vi "VISA_ReadAndSave_8CHparalelos COM BUFFER DE LEITURA.vi"() -> ()   [LabVIEW 2019]
uses:
  813f916b-c519-439e-9418-14bd48b6d342.vi
  <vilib>/Instr/_visa.llb/VISA Configure Serial Port (Instr).vi
  <vilib>/Analysis/Matrix/Comparison/Not Equal/Not Equal.vi
  <vilib>/Analysis/Matrix/Comparison/Not Equal/Not Equal - RM,RM.vi
panel:
  in  "Tamanho do Buffer (leitura/plot)":i32=10
  out "loop time (ms)":dbl format="%.2f"
  out "Plot 7":dbl[](graph)
  out "Plot 6":dbl[](graph)
  out "Plot 5":dbl[](graph)
  out "Plot 4":dbl[](graph)
  out "Plot 3":dbl[](graph)
  out "Plot 2":dbl[](graph)
  out "Status Arquivo":errorcluster
  in  "file name":string
  out "Plot 1":dbl[](graph)
  out "Plot 0":dbl[](graph)
  out "Status Leitura":errorcluster
  out "Conversão Numérica":dbl[](array[numeric])
  out "Prévia da Leitura":string
  out "Status USB":errorcluster
  in  "Salvar Registro":bool
  in  "Gravando":bool
  in  "baud rate (115200)":u32=115200 caption="baud rate (9600)"
  in  "data bits (8)":u8=8 min=5 max=8 step=1
  in  "VISA resource name":refnum<visa-resource-name>="COM3"
  # "Controle de Salvamento"
  # "Log de Erros"
  # "Conversão Para Inteiro"
  # "Resultado da Leitura"
  # "Controle da porta Serial USB"
  # "Controle da Leitura"
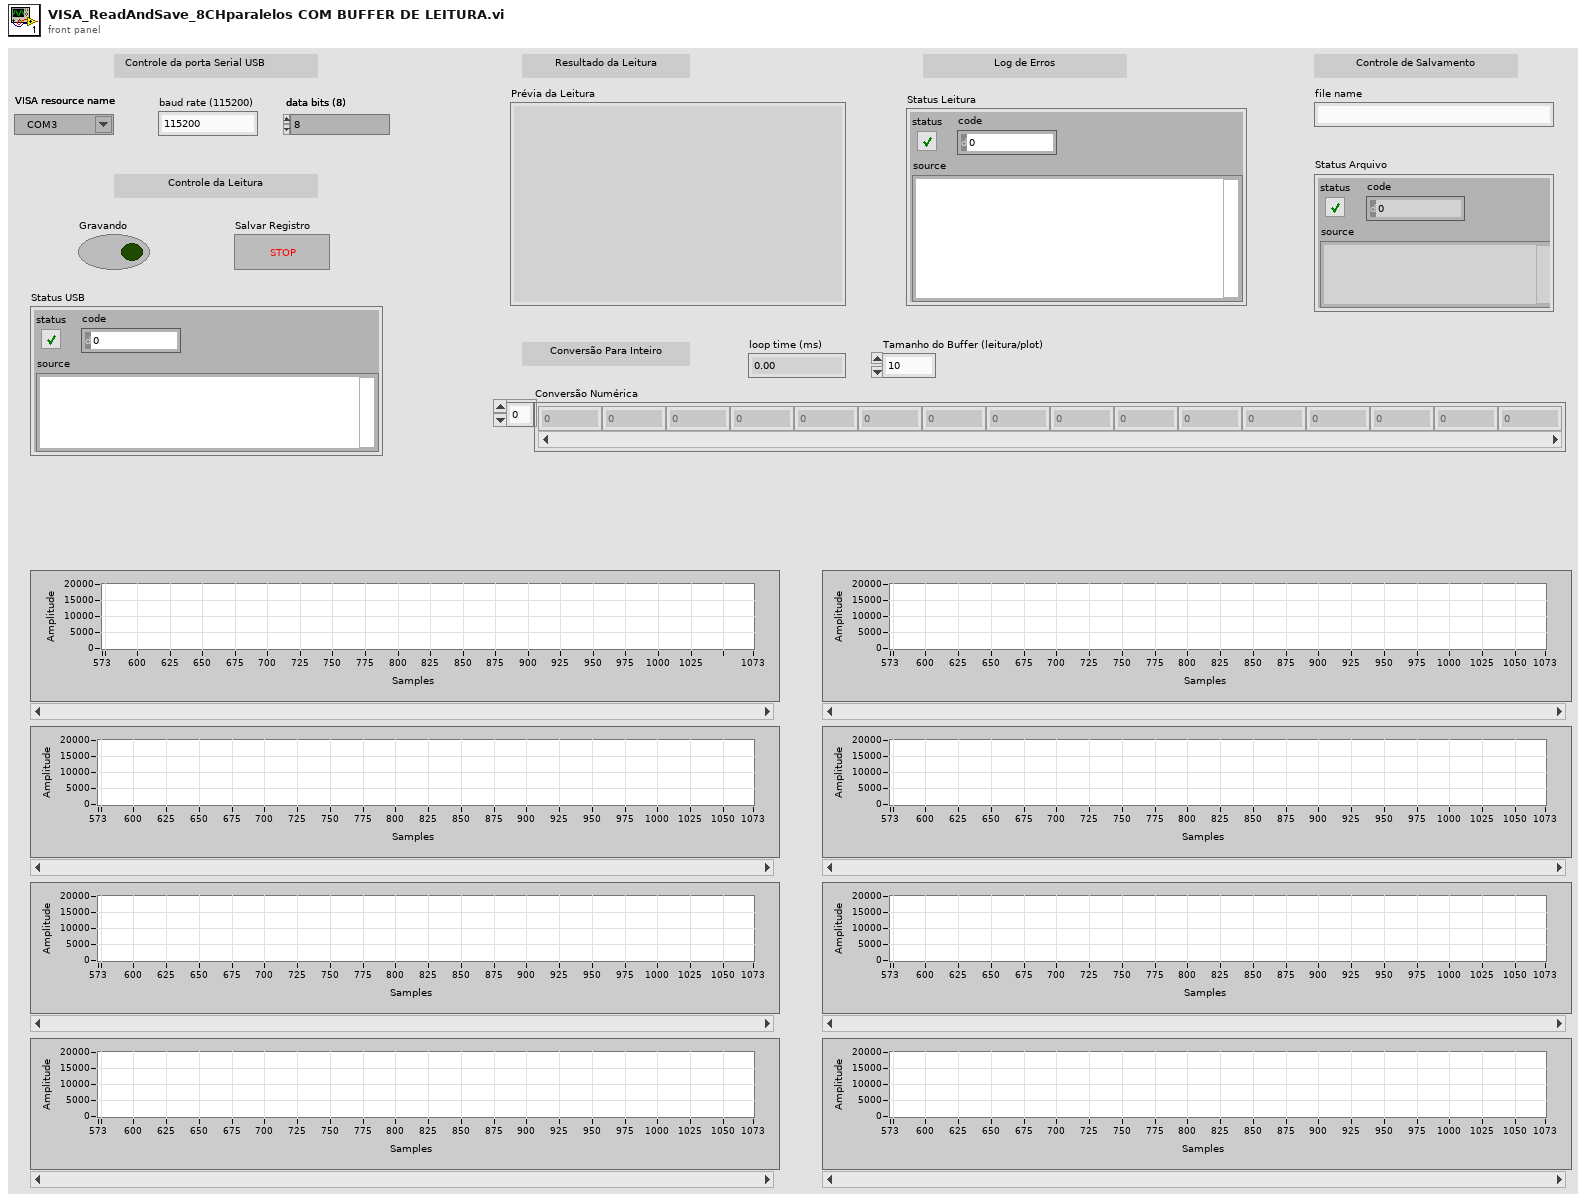
[diagram p1: front panel]
types:
  T1 = typedef "NI_Matrix.lvlib/RealMatrix.ctl" = dbl[][]
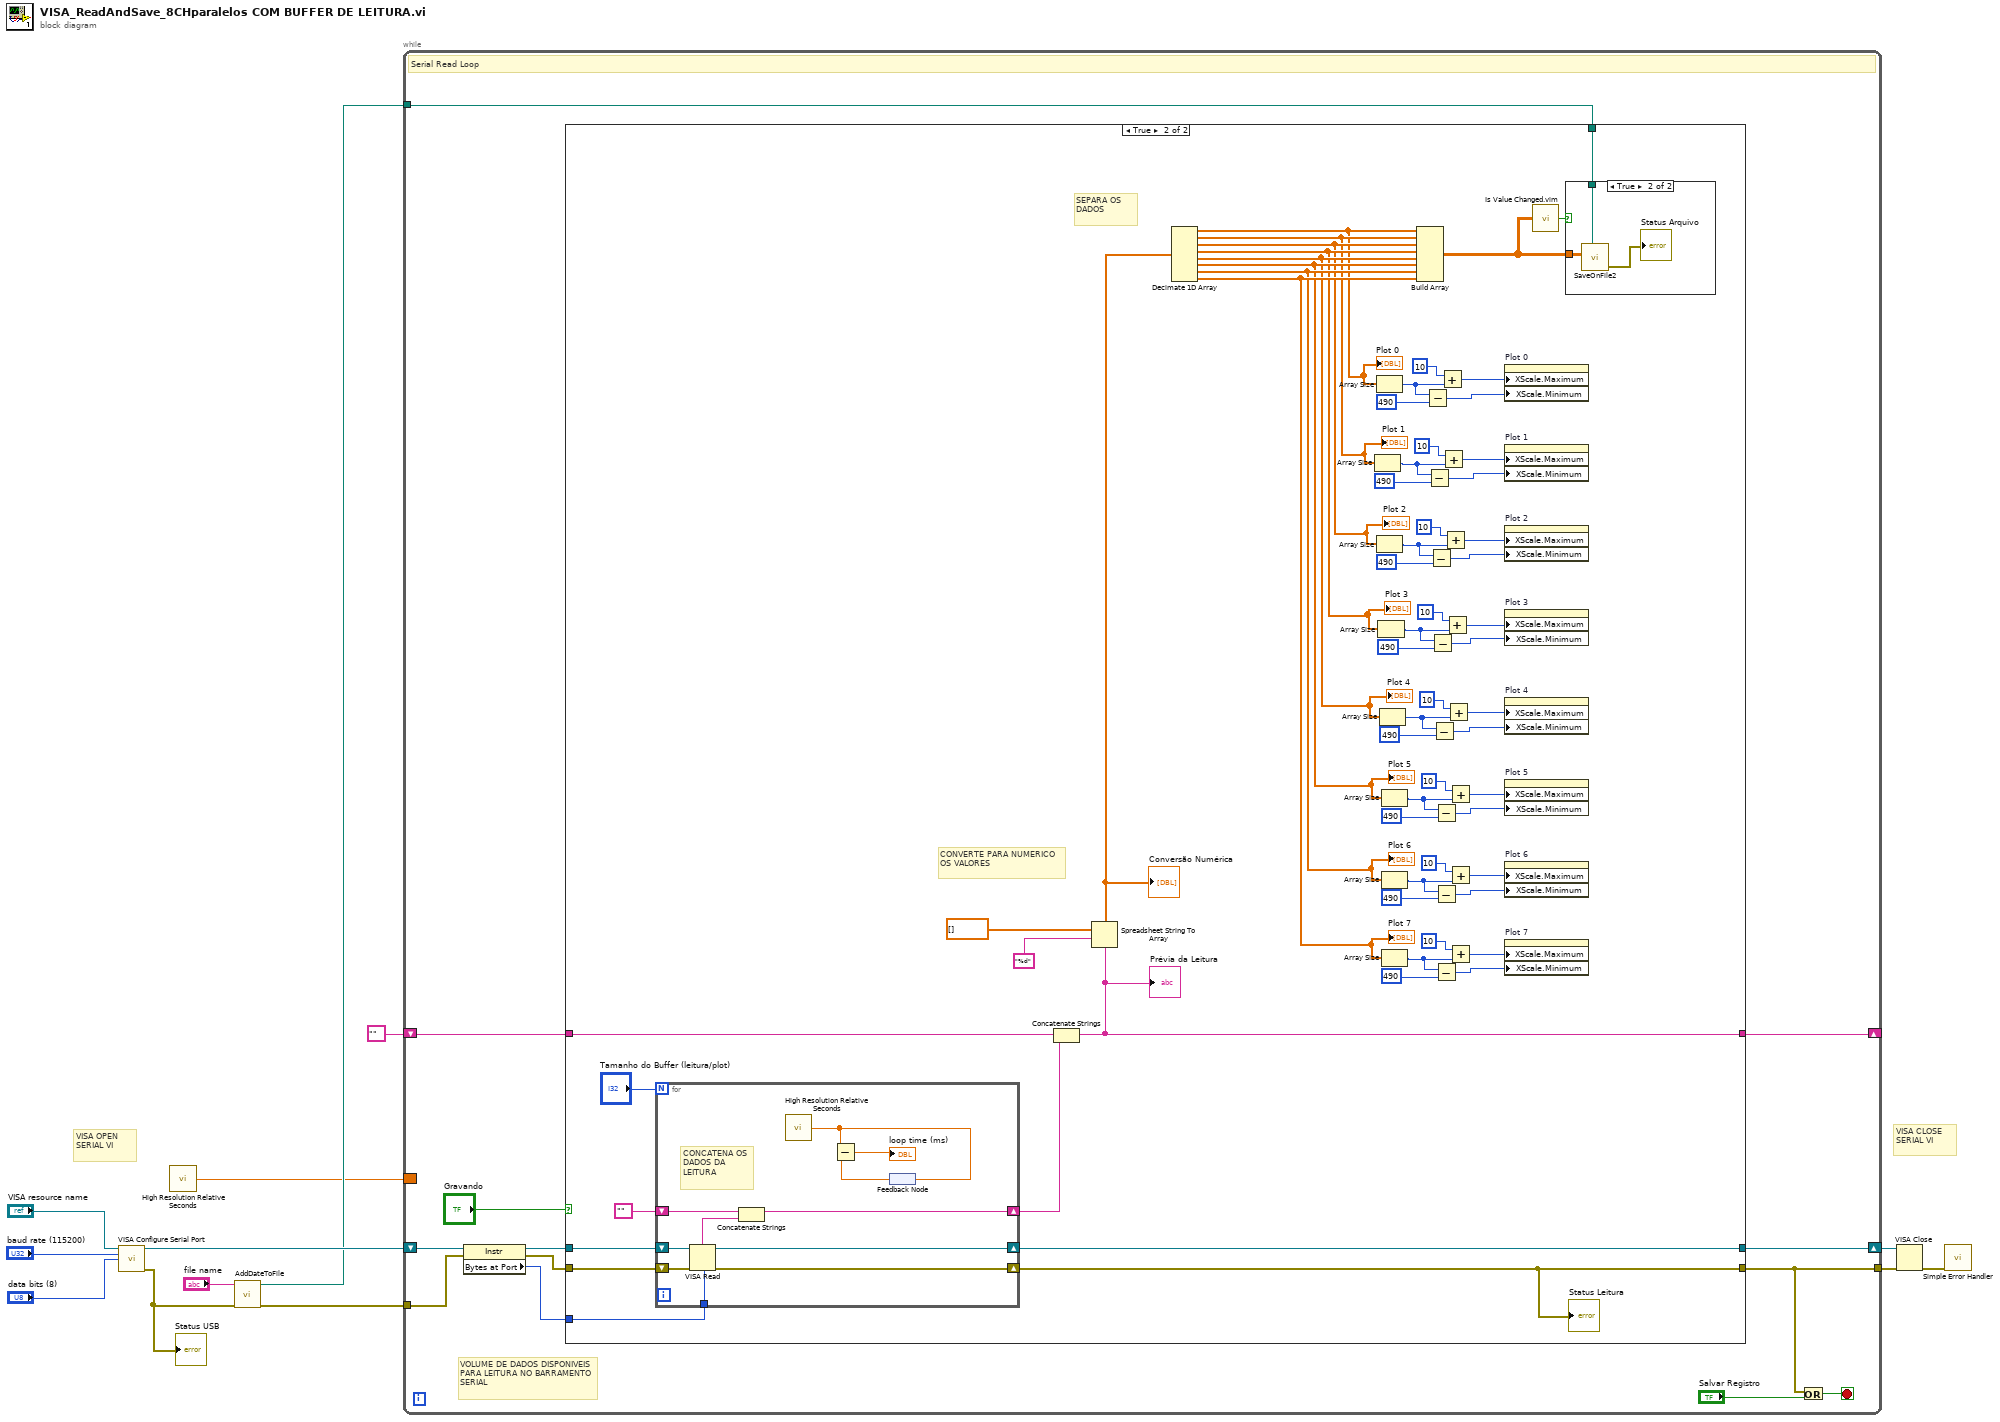
[diagram p0: block diagram]
diagram:
  # "VISA OPEN SERIAL VI"
  # "VISA CLOSE SERIAL VI"
  n1 = call-poly "VISA Configure Serial Port"("VISA resource name"="VISA resource name", "baud rate (9600)"="baud rate (115200)", "data bits (8)"="data bits (8)") -> ("VISA resource name out"=w11:refnum<visa-resource-name>, "error out"=w4:errorcluster)  [unwired: 11 in]
  "Status USB" <- w4
  n2 = call <vilib>:"High Resolution Relative Seconds.vi"() -> ("relative seconds"=w2:dbl)
  n3 = call "AddDateToFile.vi"("error in (no error)"=w4, "file name"="file name") -> ("error out"=w5:errorcluster, "new file path (Not A Path if cancelled)"=w3:path)  [unwired: 8 in]
  n4 = while {
    tunnel: w5 -> [w18]
    tunnel: [w24] -> w12
    shift-right: [w23] -> w10
    shift-left: w11 -> [w21]
    tunnel: w3 -> [w17]
    shift-right: [w15] -> _
    shift-left: "" -> [w16]
    border: w2 -> [_]
    stop <- w22 stop-if-true
    # "VOLUME DE DADOS DISPONIVEIS PARA LEITURA NO BARRAMENTO SERIAL"
    # "Serial Read Loop"
    n5 = property class="Instr"(reference=w21, error in=w18) -> (reference out=w19:refnum<visa-resource-name>, error out=w20:errorcluster, "Bytes at Port"=w14:u32)
    n6 = case shown="True" "Gravando" {
      tunnel: [w28 w35] -> w24
      tunnel: [w29 w34] -> w23
      tunnel: w19 -> [w29 w37]
      tunnel: w20 -> [w28 w36]
      tunnel: w17 -> [_ w85]
      tunnel: w16 -> [w27 w38]
      tunnel: [w27 w33] -> w15
      tunnel: w14 -> [_ w31]
      frame False {
        # "OS DADOS SÃO ACUMULADOS NO BUFFER ESPERANDO A PERMISSÃO PARA SER LIDOS"
      }
      frame True {
        # "SEPARA OS DADOS"
        # "CONVERTE PARA NUMERICO OS VALORES"
        n7 = for {
          N: "Tamanho do Buffer (leitura/plot)" -> [_]
          shift-right: [w103] -> w39
          shift-left: "" -> [w104]
          shift-right: [w99] -> w35
          shift-left: w36 -> [w100]
          shift-right: [w98] -> w34
          shift-left: w37 -> [w101]
          tunnel: w31 -> [w97]
          # "CONCATENA OS DADOS DA LEITURA"
          n8 = VISA Read(VISA resource name=w101, byte count=w97, error in (no error)=w100) -> (VISA resource name out=w98:refnum<visa-resource-name>, read buffer=w102:string, error out=w99:errorcluster)  [unwired: 1 out]
          n9 = Concatenate Strings(w104, w102) -> (w103:string)
          n10 = call <vilib>:"High Resolution Relative Seconds.vi"() -> ("relative seconds"=w95:dbl)
          n11 = feedback #1() -> (w94:dbl)
          n12 = Subtract(x=w95, y=w94) -> (x-y=→"loop time (ms)":dbl)
          n13 = feedback-in #1(w95) -> ()
        }
        "Status Leitura" <- w35
        n14 = Concatenate Strings(w38, w39) -> (w33:string)
        "Prévia da Leitura" <- w33
        n15 = Spreadsheet String To Array(format string="%d", spreadsheet string=w33, array type (2D Dbl)=dbl[] []) -> (array=w41:dbl[])  [unwired: 1 in]
        "Conversão Numérica" <- w41
        n16 = Decimate 1D Array(w41) -> (w42:dbl[], w43:dbl[], w44:dbl[], w45:dbl[], w46:dbl[], w47:dbl[], w48:dbl[], w49:dbl[])
        "Plot 0" <- w42
        "Plot 1" <- w43
        "Plot 2" <- w44
        "Plot 3" <- w45
        "Plot 4" <- w46
        "Plot 5" <- w47
        "Plot 6" <- w48
        "Plot 7" <- w49
        n17 = Array Size(array=w43) -> (size(s)=w81:i32)
        n18 = Array Size(array=w42) -> (size(s)=w88:i32)
        n19 = Array Size(array=w44) -> (size(s)=w78:i32)
        n20 = Array Size(array=w45) -> (size(s)=w75:i32)
        n21 = Array Size(array=w46) -> (size(s)=w72:i32)
        n22 = Array Size(array=w47) -> (size(s)=w69:i32)
        n23 = Array Size(array=w48) -> (size(s)=w66:i32)
        n24 = Array Size(array=w49) -> (size(s)=w63:i32)
        n25 = Build Array(w42, w43, w44, w45, w46, w47, w48, w49) -> (w32:T1)
        n26 = Subtract(x=w88, y=490) -> (x-y=w89:i32)
        n27 = Subtract(x=w81, y=490) -> (x-y=w84:i32)
        n28 = Subtract(x=w78, y=490) -> (x-y=w60:i32)
        n29 = Subtract(x=w75, y=490) -> (x-y=w58:i32)
        n30 = Subtract(x=w72, y=490) -> (x-y=w53:i32)
        n31 = Subtract(x=w69, y=490) -> (x-y=w52:i32)
        n32 = Subtract(x=w66, y=490) -> (x-y=w51:i32)
        n33 = Subtract(x=w63, y=490) -> (x-y=w50:i32)
        n34 = Add(x=10, y=w88) -> (x+y=w87:i32)
        n35 = Add(x=10, y=w81) -> (x+y=w83:i32)
        n36 = Add(x=10, y=w78) -> (x+y=w61:i32)
        n37 = Add(x=10, y=w75) -> (x+y=w59:i32)
        n38 = Add(x=10, y=w72) -> (x+y=w57:i32)
        n39 = Add(x=10, y=w69) -> (x+y=w56:i32)
        n40 = Add(x=10, y=w66) -> (x+y=w55:i32)
        n41 = Add(x=10, y=w63) -> (x+y=w54:i32)
        n42 = property on="Plot 0" class="WFGraph (strict)"("XScale.Maximum"=w87, "XScale.Minimum"=w89) -> ()  [unwired: 2 in, 2 out]
        n43 = property on="Plot 1" class="WFGraph (strict)"("XScale.Maximum"=w83, "XScale.Minimum"=w84) -> ()  [unwired: 2 in, 2 out]
        n44 = property on="Plot 2" class="WFGraph (strict)"("XScale.Maximum"=w61, "XScale.Minimum"=w60) -> ()  [unwired: 2 in, 2 out]
        n45 = property on="Plot 3" class="WFGraph (strict)"("XScale.Maximum"=w59, "XScale.Minimum"=w58) -> ()  [unwired: 2 in, 2 out]
        n46 = property on="Plot 4" class="WFGraph (strict)"("XScale.Maximum"=w57, "XScale.Minimum"=w53) -> ()  [unwired: 2 in, 2 out]
        n47 = property on="Plot 5" class="WFGraph (strict)"("XScale.Maximum"=w56, "XScale.Minimum"=w52) -> ()  [unwired: 2 in, 2 out]
        n48 = property on="Plot 6" class="WFGraph (strict)"("XScale.Maximum"=w55, "XScale.Minimum"=w51) -> ()  [unwired: 2 in, 2 out]
        n49 = property on="Plot 7" class="WFGraph (strict)"("XScale.Maximum"=w54, "XScale.Minimum"=w50) -> ()  [unwired: 2 in, 2 out]
        n50 = call "Is Value Changed.vim"("value"=w32) -> ("changed or first call?"=w91:bool)
        n51 = case shown="True" w91 {
          tunnel: w32 -> [_ w105]
          tunnel: w85 -> [_ w107]
          frame False {
          }
          frame True {
            n52 = call "SaveOnFile2.vi"("2D data"=w105, "file path (dialog if empty)"=w107) -> ("error file"=→"Status Arquivo":errorcluster)  [unwired: 5 in]
          }
        }
      }
    }
    n53 = Or(x=w24, y="Salvar Registro") -> (x .or. y?=w22:bool)
  }
  n54 = VISA Close(VISA resource name=w10, error in (no error)=w12) -> (error out=w9:errorcluster)
  n55 = call <vilib>:"Simple Error Handler.vi"("error in (no error)"=w9) -> ()  [unwired: 4 in, 5 out]
